vi "Search for VISA.vi"() -> ()   [LabVIEW 2011]
panel:
  in  "VISA resource name 2":refnum<visa-resource-name>
  in  "VISA resource name":refnum<visa-resource-name>
  out "Array":T1(array[cluster])
  out "find list":string[](array[string])
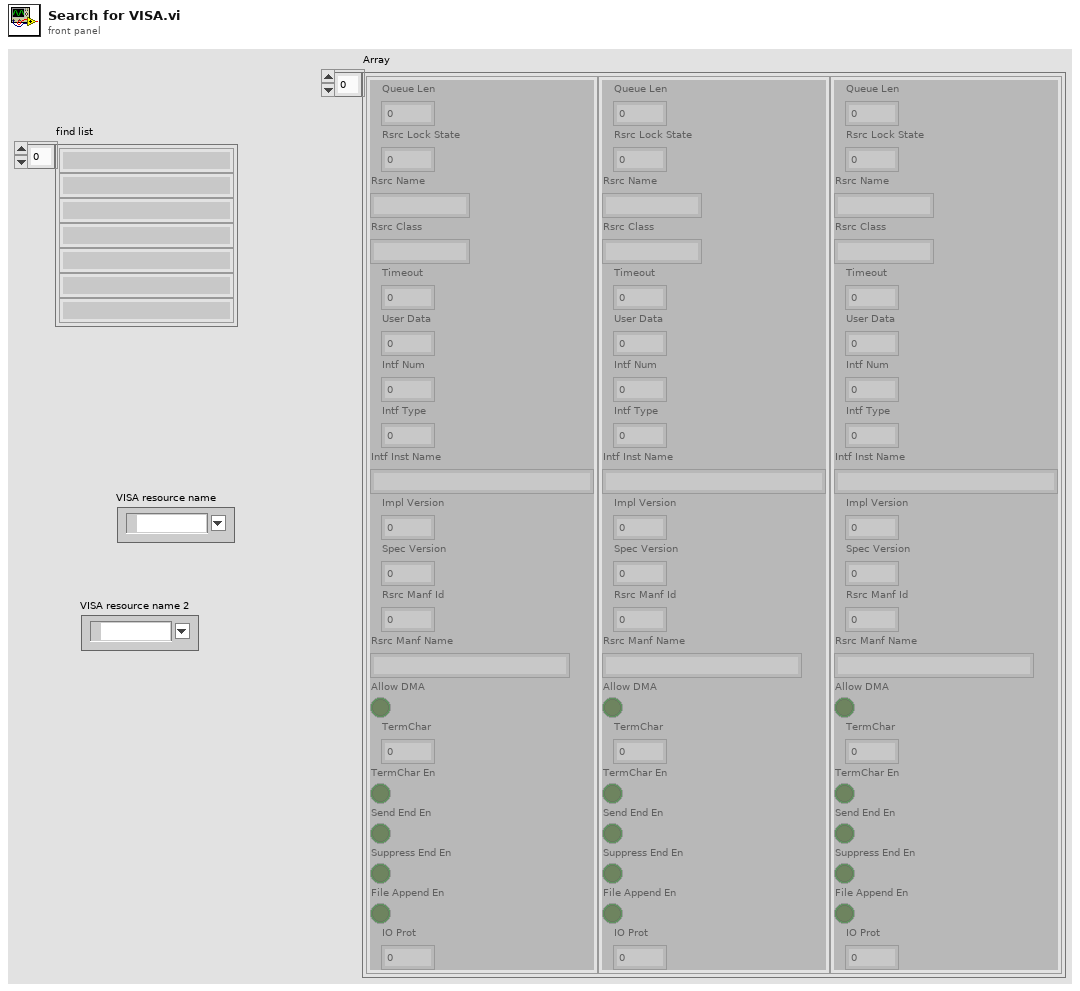
[diagram p1: front panel]
types:
  T1 = cluster{"Queue Len":u32, "Rsrc Lock State":u32, "Rsrc Name":string, "Rsrc Class":string, "Timeout":u32, "User Data":u32, "Intf Num":u16, "Intf Type":u16, "Intf Inst Name":string, "Impl Version":u32, "Spec Version":u32, "Rsrc Manf Id":u16, "Rsrc Manf Name":string, "Allow DMA":bool, "TermChar":u8, "TermChar En":bool, "Send End En":bool, "Suppress End En":bool, "File Append En":bool, "IO Prot":u16}[]
  T2 = cluster{"Queue Len":u32, "Rsrc Lock State":u32, "Rsrc Name":string, "Rsrc Class":string, "Timeout":u32, "User Data":u32, "Intf Num":u16, "Intf Type":u16, "Intf Inst Name":string, "Impl Version":u32, "Spec Version":u32, "Rsrc Manf Id":u16, "Rsrc Manf Name":string, "Allow DMA":bool, "TermChar":u8, "TermChar En":bool, "Send End En":bool, "Suppress End En":bool, "File Append En":bool, "IO Prot":u16}
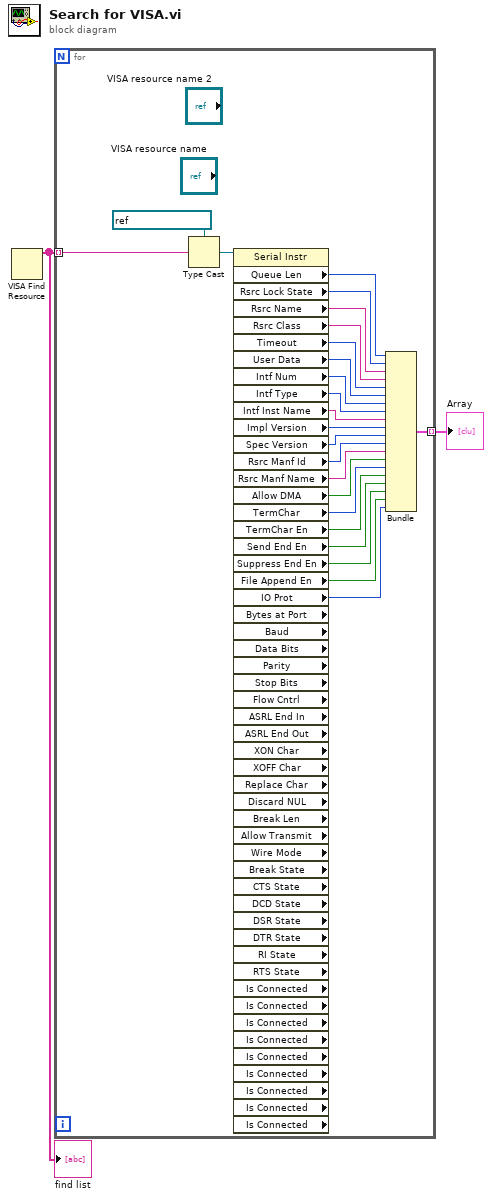
[diagram p0: block diagram]
diagram:
  n1 = VISA Find Resource() -> (3:w2:string[])  [unwired: 3 in, 2 out]
  "find list" <- w2
  n2 = for {
    tunnel: w2 -> [w25] mode=indexing
    tunnel: [w23] -> w1 mode=indexing
    n3 = Type Cast(type=refnum<visa-resource-name> "ASRL3::INSTR" ("VISA resource name"), x=w25) -> (*(type *) &x=w24:refnum<visa-resource-name>)
    n4 = property class="Serial Instr" props=["Queue Len", "Rsrc Lock State", "Rsrc Name", "Rsrc Class", "Timeout", "User Data", "Intf Num", "Intf Type", "Intf Inst Name", "Impl Version", "Spec Version", "Rsrc Manf Id", "Rsrc Manf Name", "Allow DMA", "TermChar", "TermChar En", "Send End En", "Suppress End En", "File Append En", "IO Prot", "Bytes at Port", "Baud", "Data Bits", "Parity", "Stop Bits", "Flow Cntrl", "ASRL End In", "ASRL End Out", "XON Char", "XOFF Char", "Replace Char", "Discard NUL", "Break Len", "Allow Transmit", "Wire Mode", "Break State", "CTS State", "DCD State", "DSR State", "DTR State", "RI State", "RTS State", "Is Connected", "Is Connected", "Is Connected", "Is Connected", "Is Connected", "Is Connected", "Is Connected", "Is Connected", "Is Connected"](reference=w24) -> ("Queue Len"=w22:u32, "Rsrc Lock State"=w21:u32, "Rsrc Name"=w20:string, "Rsrc Class"=w19:string, "Timeout"=w18:u32, "User Data"=w17:u32, "Intf Num"=w16:u16, "Intf Type"=w15:u16, "Intf Inst Name"=w14:string, "Impl Version"=w13:u32, "Spec Version"=w12:u32, "Rsrc Manf Id"=w11:u16, "Rsrc Manf Name"=w10:string, "Allow DMA"=w9:bool, "TermChar"=w8:u8, "TermChar En"=w7:bool, "Send End En"=w6:bool, "Suppress End En"=w5:bool, "File Append En"=w4:bool, "IO Prot"=w3:u16)  [unwired: 1 in, 33 out]
    n5 = Bundle("Queue Len"=w22, "Rsrc Lock State"=w21, "Rsrc Name"=w20, "Rsrc Class"=w19, "Timeout"=w18, "User Data"=w17, "Intf Num"=w16, "Intf Type"=w15, "Intf Inst Name"=w14, "Impl Version"=w13, "Spec Version"=w12, "Rsrc Manf Id"=w11, "Rsrc Manf Name"=w10, "Allow DMA"=w9, "TermChar"=w8, "TermChar En"=w7, "Send End En"=w6, "Suppress End En"=w5, "File Append En"=w4, "IO Prot"=w3) -> (w23:T2)  [unwired: 1 in]
  }
  "Array" <- w1
